vi "guangzi.vi"() -> ()   [LabVIEW 2016]
uses:
  <vilib>/Utility/file.llb/Write To Spreadsheet File (DBL).vi
panel:
  out "切片图":u32[](graph)
  in  "切片值":i32
  in  "选项卡控件":T1(tab)
  in  "对数":bool
  out "MCS8Dat Error":i32
  out "CHN Status":T2 {"Dummy" format="%.2f"; "Starts" format="%.2f"; "Sweeps" format="%.2f"; "Roirate" format="%.2f"; "RoiSum" format="%.2f"; "TotalSum" format="%.2f"; "Fifo full" format="%.2f"; "Runtime" format="%.2f"}
  out "Data":u32[](graph)
  out "Settings":T3 {"dummy3" format="%.2f"; "dummy2" format="%.2f"; "bitshift" format="%.0x"; "Active" format="%.0x"; "Offset" format="%.0x"; "Param" format="%.0x"; "dummy1" format="%.2f"; "Roipreset" format="%.2f"; "cftfak" format="%.0x"}
  out "通道数":i32
  out "Data 9":dbl[](graph)
  out "Data 2":u32[](graph)
  out "MCS8Dat Error 2":i32
  out "Settings 2":T3 {"dummy3" format="%.2f"; "dummy2" format="%.2f"; "bitshift" format="%.0x"; "Active" format="%.0x"; "Offset" format="%.0x"; "Param" format="%.0x"; "dummy1" format="%.2f"; "Roipreset" format="%.2f"; "cftfak" format="%.0x"}
  out "CHN Status 2":T2 {"Dummy" format="%.2f"; "Starts" format="%.2f"; "Sweeps" format="%.2f"; "Roirate" format="%.2f"; "RoiSum" format="%.2f"; "TotalSum" format="%.2f"; "Fifo full" format="%.2f"; "Runtime" format="%.2f"}
  out "通道数 2":i32
  in  "对数 2":bool
  out "Data10":dbl[](graph)
  out "Data 3":u32[](graph)
  out "MCS8Dat Error 3":i32
  out "Settings 3":T3 {"dummy3" format="%.2f"; "dummy2" format="%.2f"; "bitshift" format="%.0x"; "Active" format="%.0x"; "Offset" format="%.0x"; "Param" format="%.0x"; "dummy1" format="%.2f"; "Roipreset" format="%.2f"; "cftfak" format="%.0x"}
  out "CHN Status 3":T2 {"Dummy" format="%.2f"; "Starts" format="%.2f"; "Sweeps" format="%.2f"; "Roirate" format="%.2f"; "RoiSum" format="%.2f"; "TotalSum" format="%.2f"; "Fifo full" format="%.2f"; "Runtime" format="%.2f"}
  out "通道数 3":i32
  in  "对数 3":bool
  out "Data10 2":dbl[](graph)
  out "Data 4":u32[](graph)
  out "MCS8Dat Error 4":i32
  out "Settings 4":T3 {"dummy3" format="%.2f"; "dummy2" format="%.2f"; "bitshift" format="%.0x"; "Active" format="%.0x"; "Offset" format="%.0x"; "Param" format="%.0x"; "dummy1" format="%.2f"; "Roipreset" format="%.2f"; "cftfak" format="%.0x"}
  out "CHN Status 4":T2 {"Dummy" format="%.2f"; "Starts" format="%.2f"; "Sweeps" format="%.2f"; "Roirate" format="%.2f"; "RoiSum" format="%.2f"; "TotalSum" format="%.2f"; "Fifo full" format="%.2f"; "Runtime" format="%.2f"}
  out "通道数 4":i32
  in  "对数 4":bool
  out "Data10 3":dbl[](graph)
  out "Data 5":u32[](graph)
  out "MCS8Dat Error 5":i32
  out "Settings 5":T3 {"dummy3" format="%.2f"; "dummy2" format="%.2f"; "bitshift" format="%.0x"; "Active" format="%.0x"; "Offset" format="%.0x"; "Param" format="%.0x"; "dummy1" format="%.2f"; "Roipreset" format="%.2f"; "cftfak" format="%.0x"}
  out "CHN Status 5":T2 {"Dummy" format="%.2f"; "Starts" format="%.2f"; "Sweeps" format="%.2f"; "Roirate" format="%.2f"; "RoiSum" format="%.2f"; "TotalSum" format="%.2f"; "Fifo full" format="%.2f"; "Runtime" format="%.2f"}
  out "通道数 5":i32
  in  "对数 5":bool
  out "Data10 4":dbl[](graph)
  out "Data 6":u32[](graph)
  out "MCS8Dat Error 6":i32
  out "Settings 6":T3 {"dummy3" format="%.2f"; "dummy2" format="%.2f"; "bitshift" format="%.0x"; "Active" format="%.0x"; "Offset" format="%.0x"; "Param" format="%.0x"; "dummy1" format="%.2f"; "Roipreset" format="%.2f"; "cftfak" format="%.0x"}
  out "CHN Status 6":T2 {"Dummy" format="%.2f"; "Starts" format="%.2f"; "Sweeps" format="%.2f"; "Roirate" format="%.2f"; "RoiSum" format="%.2f"; "TotalSum" format="%.2f"; "Fifo full" format="%.2f"; "Runtime" format="%.2f"}
  out "通道数 6":i32
  in  "对数 6":bool
  out "Data10 5":dbl[](graph)
  out "Data 7":u32[](graph)
  out "MCS8Dat Error 7":i32
  out "Settings 7":T3 {"dummy3" format="%.2f"; "dummy2" format="%.2f"; "bitshift" format="%.0x"; "Active" format="%.0x"; "Offset" format="%.0x"; "Param" format="%.0x"; "dummy1" format="%.2f"; "Roipreset" format="%.2f"; "cftfak" format="%.0x"}
  out "CHN Status 7":T2 {"Dummy" format="%.2f"; "Starts" format="%.2f"; "Sweeps" format="%.2f"; "Roirate" format="%.2f"; "RoiSum" format="%.2f"; "TotalSum" format="%.2f"; "Fifo full" format="%.2f"; "Runtime" format="%.2f"}
  out "通道数 7":i32
  in  "对数 7":bool
  out "Data10 6":dbl[](graph)
  out "Data 8":u32[](graph)
  out "MCS8Dat Error 8":i32
  out "Settings 8":T3 {"dummy3" format="%.2f"; "dummy2" format="%.2f"; "bitshift" format="%.0x"; "Active" format="%.0x"; "Offset" format="%.0x"; "Param" format="%.0x"; "dummy1" format="%.2f"; "Roipreset" format="%.2f"; "cftfak" format="%.0x"}
  out "CHN Status 8":T2 {"Dummy" format="%.2f"; "Starts" format="%.2f"; "Sweeps" format="%.2f"; "Roirate" format="%.2f"; "RoiSum" format="%.2f"; "TotalSum" format="%.2f"; "Fifo full" format="%.2f"; "Runtime" format="%.2f"}
  out "通道数 8":i32
  in  "对数 8":bool
  out "Data10 7":dbl[](graph)
  in  "子开关":bool
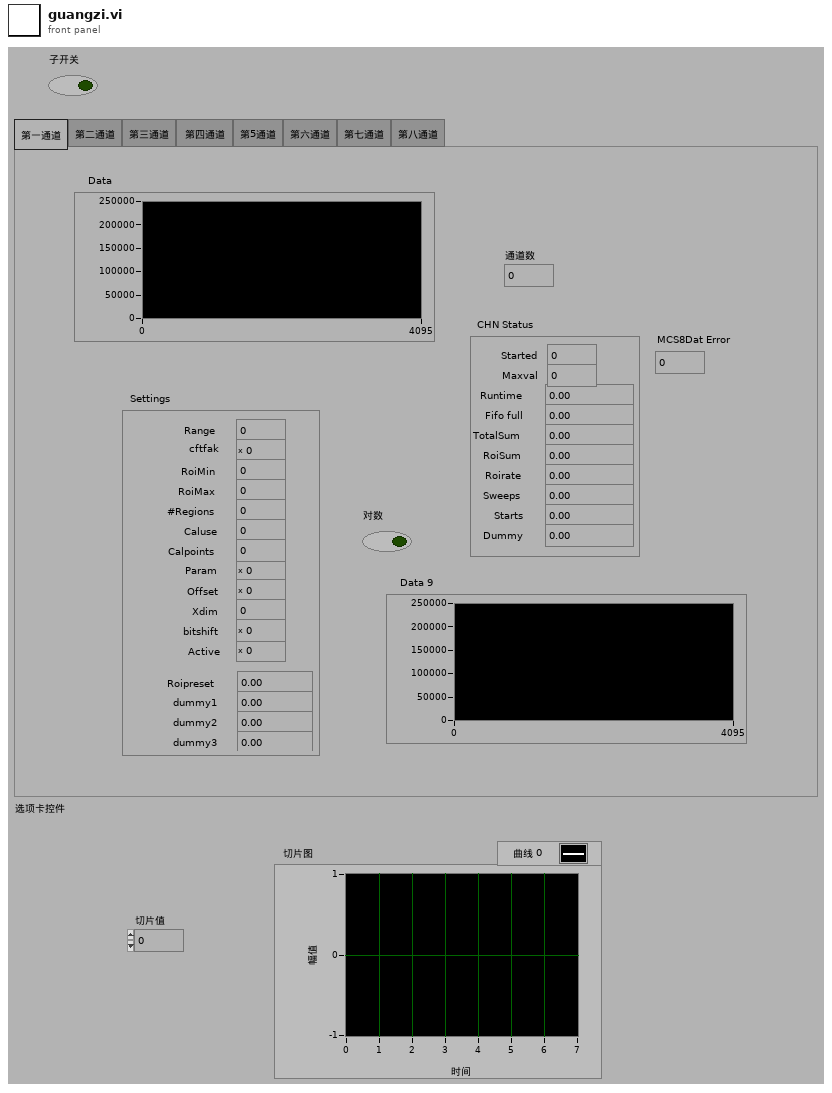
[diagram p1: front panel]
types:
  T1 = enum32{"第一通道", "第二通道", "第三通道", "第四通道 ", "第5通道", "第六通道", "第七通道", "第八通道"}
  T2 = cluster{"Started":i32, "Maxval":u32, "Runtime":dbl, "Fifo full":dbl, "TotalSum":dbl, "RoiSum":dbl, "Roirate":dbl, "Sweeps":dbl, "Starts":dbl, "Dummy":dbl}
  T3 = cluster{"Range":i32, "cftfak":i32, "RoiMin":i32, "RoiMax":i32, "#Regions":i32, "Caluse":i32, "Calpoints":i32, "Param":i32, "Offset":i32, "Xdim":i32, "bitshift":i32, "Active":i32, "Roipreset":dbl, "dummy1":dbl, "dummy2":dbl, "dummy3":dbl}
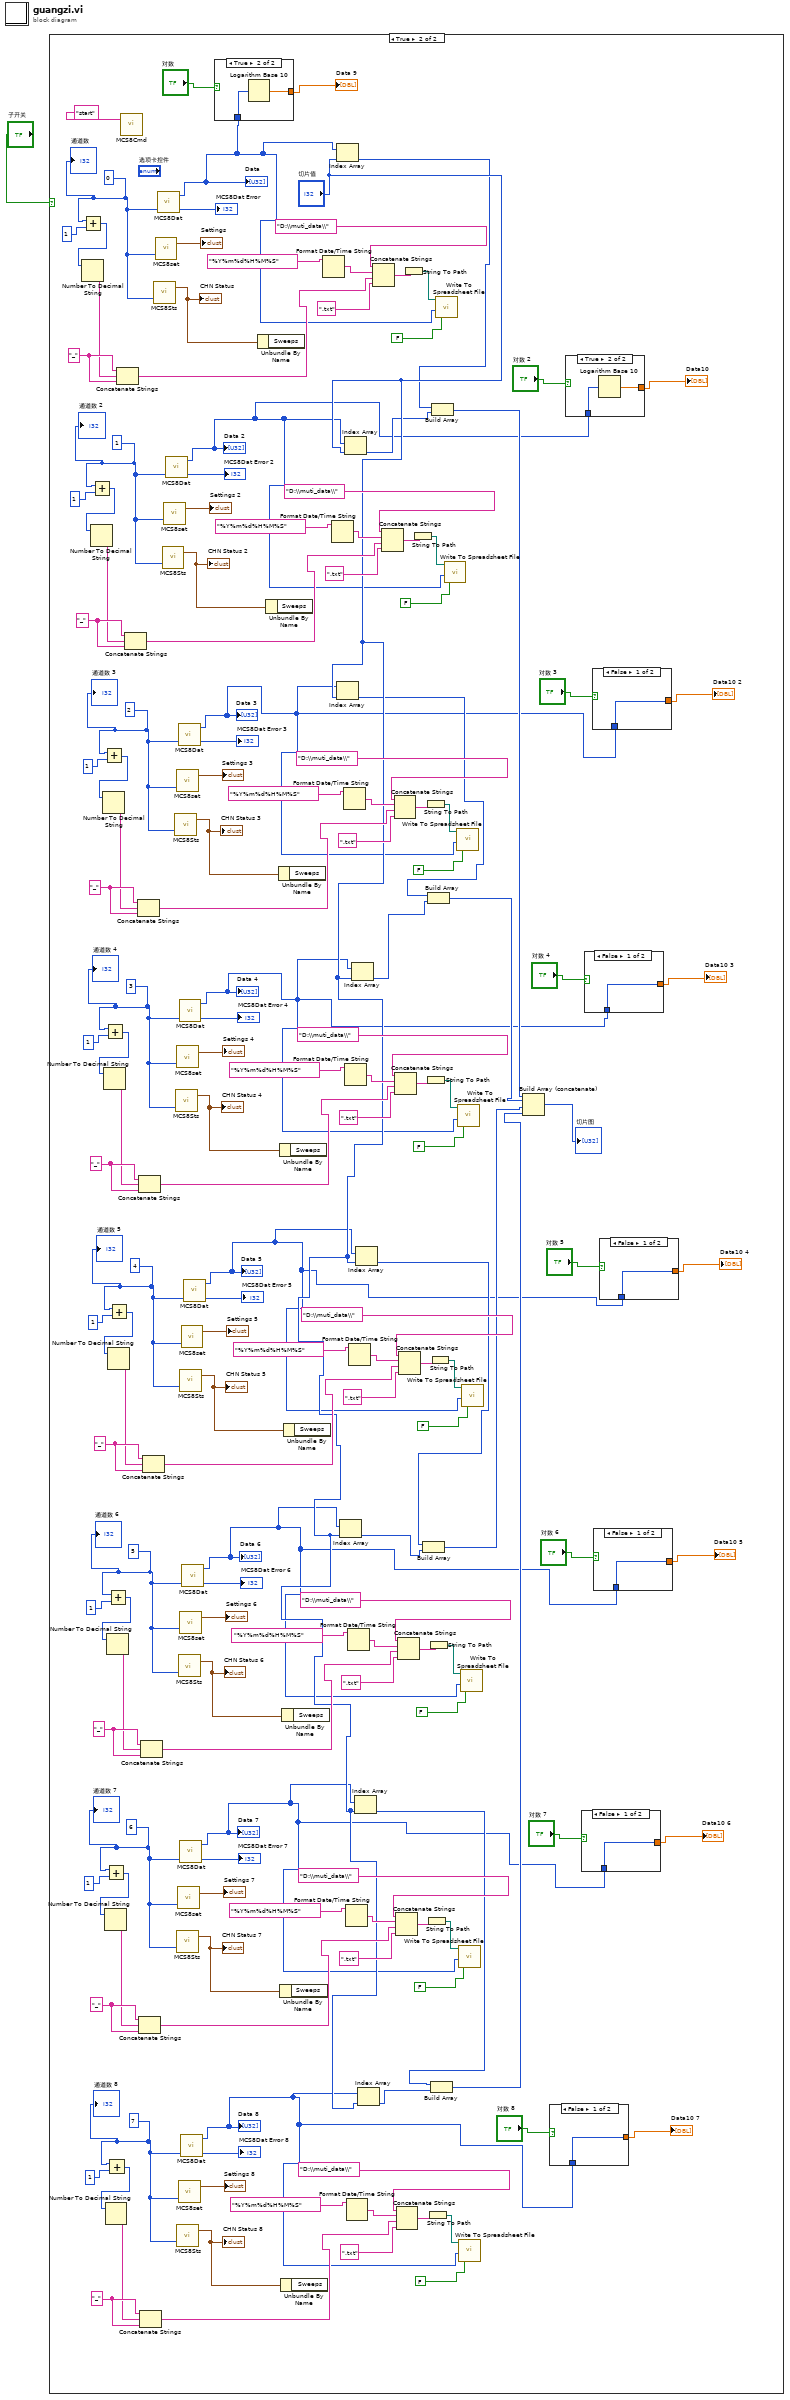
[diagram p0: block diagram]
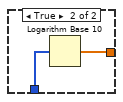
[diagram p3: hidden frame]
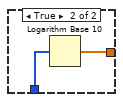
[diagram p4: hidden frame]
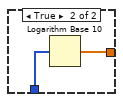
[diagram p5: hidden frame]
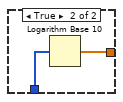
[diagram p6: hidden frame]
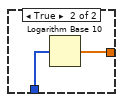
[diagram p7: hidden frame]
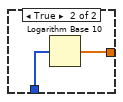
[diagram p8: hidden frame]
diagram:
  n1 = case shown="True" "子开关" {
    frame False {
    }
    frame True {
      w40 = 7
      w49 = "_"
      w56 = 6
      w65 = "_"
      w72 = 5
      w81 = "_"
      w88 = 4
      w97 = "_"
      w104 = 3
      w113 = "_"
      w120 = 2
      w129 = "_"
      w136 = 1
      w145 = "_"
      w152 = 0
      w161 = "_"
      n2 = Add(x=w152, y=1) -> (x+y=w155:i32)
      n3 = Number To Decimal String(number=w155) -> (decimal integer string=w160:string)  [unwired: 1 in]
      n4 = Add(x=w136, y=1) -> (x+y=w139:i32)
      n5 = Number To Decimal String(number=w139) -> (decimal integer string=w144:string)  [unwired: 1 in]
      n6 = Add(x=w120, y=1) -> (x+y=w123:i32)
      n7 = Number To Decimal String(number=w123) -> (decimal integer string=w128:string)  [unwired: 1 in]
      n8 = Add(x=w104, y=1) -> (x+y=w107:i32)
      n9 = Number To Decimal String(number=w107) -> (decimal integer string=w112:string)  [unwired: 1 in]
      n10 = Add(x=w56, y=1) -> (x+y=w59:i32)
      n11 = Number To Decimal String(number=w59) -> (decimal integer string=w64:string)  [unwired: 1 in]
      n12 = Add(x=w40, y=1) -> (x+y=w43:i32)
      n13 = Number To Decimal String(number=w43) -> (decimal integer string=w48:string)  [unwired: 1 in]
      n14 = Add(x=w72, y=1) -> (x+y=w75:i32)
      n15 = Number To Decimal String(number=w75) -> (decimal integer string=w80:string)  [unwired: 1 in]
      n16 = Add(x=w88, y=1) -> (x+y=w91:i32)
      n17 = Number To Decimal String(number=w91) -> (decimal integer string=w96:string)  [unwired: 1 in]
      n18 = Concatenate Strings(w161, w160, w161) -> (w159:string)
      n19 = call "MCS8Cmd.vi"("Command"="start") -> ()  [unwired: 2 in, 1 out]
      n20 = Concatenate Strings(w145, w144, w145) -> (w143:string)
      n21 = Concatenate Strings(w129, w128, w129) -> (w127:string)
      n22 = Concatenate Strings(w113, w112, w113) -> (w111:string)
      n23 = Concatenate Strings(w65, w64, w65) -> (w63:string)
      n24 = Concatenate Strings(w49, w48, w49) -> (w47:string)
      n25 = Concatenate Strings(w81, w80, w81) -> (w79:string)
      n26 = Concatenate Strings(w97, w96, w97) -> (w95:string)
      n27 = call "MCS8Sts.vi"("CHN #"=w152) -> ("CHN Status"=w167:T2)  [unwired: 1 in, 1 out]
      "CHN Status" <- w167
      n28 = call "MCS8set.vi"("Spect #"=w152) -> ("Settings"=→"Settings":T3)  [unwired: 1 in, 1 out]
      n29 = call "MCS8Dat.vi"("Spectrum #"=w152) -> ("MCS8Dat Error"=→"MCS8Dat Error":i32, "Data"=w24:u32[])  [unwired: 2 in, 1 out]
      "Data" <- w24
      n30 = call "MCS8Sts.vi"("CHN #"=w136) -> ("CHN Status"=w151:T2)  [unwired: 1 in, 1 out]
      "CHN Status 2" <- w151
      n31 = call "MCS8set.vi"("Spect #"=w136) -> ("Settings"=→"Settings 2":T3)  [unwired: 1 in, 1 out]
      n32 = call "MCS8Dat.vi"("Spectrum #"=w136) -> ("MCS8Dat Error"=→"MCS8Dat Error 2":i32, "Data"=w20:u32[])  [unwired: 2 in, 1 out]
      "Data 2" <- w20
      n33 = call "MCS8Sts.vi"("CHN #"=w120) -> ("CHN Status"=w135:T2)  [unwired: 1 in, 1 out]
      "CHN Status 3" <- w135
      n34 = call "MCS8Sts.vi"("CHN #"=w104) -> ("CHN Status"=w119:T2)  [unwired: 1 in, 1 out]
      "CHN Status 4" <- w119
      n35 = call "MCS8set.vi"("Spect #"=w120) -> ("Settings"=→"Settings 3":T3)  [unwired: 1 in, 1 out]
      n36 = call "MCS8Sts.vi"("CHN #"=w56) -> ("CHN Status"=w71:T2)  [unwired: 1 in, 1 out]
      "CHN Status 7" <- w71
      n37 = call "MCS8set.vi"("Spect #"=w104) -> ("Settings"=→"Settings 4":T3)  [unwired: 1 in, 1 out]
      n38 = call "MCS8Sts.vi"("CHN #"=w40) -> ("CHN Status"=w55:T2)  [unwired: 1 in, 1 out]
      "CHN Status 8" <- w55
      n39 = call "MCS8set.vi"("Spect #"=w56) -> ("Settings"=→"Settings 7":T3)  [unwired: 1 in, 1 out]
      n40 = call "MCS8Dat.vi"("Spectrum #"=w120) -> ("MCS8Dat Error"=→"MCS8Dat Error 3":i32, "Data"=w17:u32[])  [unwired: 2 in, 1 out]
      "Data 3" <- w17
      n41 = call "MCS8Sts.vi"("CHN #"=w72) -> ("CHN Status"=w87:T2)  [unwired: 1 in, 1 out]
      "CHN Status 6" <- w87
      n42 = call "MCS8set.vi"("Spect #"=w40) -> ("Settings"=→"Settings 8":T3)  [unwired: 1 in, 1 out]
      n43 = call "MCS8Dat.vi"("Spectrum #"=w104) -> ("MCS8Dat Error"=→"MCS8Dat Error 4":i32, "Data"=w14:u32[])  [unwired: 2 in, 1 out]
      "Data 4" <- w14
      n44 = call "MCS8Sts.vi"("CHN #"=w88) -> ("CHN Status"=w103:T2)  [unwired: 1 in, 1 out]
      "CHN Status 5" <- w103
      n45 = call "MCS8set.vi"("Spect #"=w72) -> ("Settings"=→"Settings 6":T3)  [unwired: 1 in, 1 out]
      n46 = call "MCS8Dat.vi"("Spectrum #"=w56) -> ("MCS8Dat Error"=→"MCS8Dat Error 7":i32, "Data"=w5:u32[])  [unwired: 2 in, 1 out]
      "Data 7" <- w5
      n47 = call "MCS8Dat.vi"("Spectrum #"=w40) -> ("MCS8Dat Error"=→"MCS8Dat Error 8":i32, "Data"=w2:u32[])  [unwired: 2 in, 1 out]
      "Data 8" <- w2
      n48 = call "MCS8set.vi"("Spect #"=w88) -> ("Settings"=→"Settings 5":T3)  [unwired: 1 in, 1 out]
      n49 = call "MCS8Dat.vi"("Spectrum #"=w72) -> ("MCS8Dat Error"=→"MCS8Dat Error 6":i32, "Data"=w8:u32[])  [unwired: 2 in, 1 out]
      "Data 6" <- w8
      n50 = call "MCS8Dat.vi"("Spectrum #"=w88) -> ("MCS8Dat Error"=→"MCS8Dat Error 5":i32, "Data"=w11:u32[])  [unwired: 2 in, 1 out]
      "Data 5" <- w11
      n51 = case shown="True" "对数" {
        tunnel: w24 -> [w190 w192]
        tunnel: [w190 w191] -> w23
        frame False {
        }
        frame True {
          n52 = Logarithm Base 10(1:w192) -> (0:w191:dbl[])
        }
      }
      "Data 9" <- w23
      n53 = Unbundle By Name(w167) -> ()  [unwired: 1 out]
      n54 = Unbundle By Name(w151) -> ()  [unwired: 1 out]
      n55 = Unbundle By Name(w135) -> ()  [unwired: 1 out]
      n56 = Unbundle By Name(w119) -> ()  [unwired: 1 out]
      n57 = Unbundle By Name(w71) -> ()  [unwired: 1 out]
      n58 = Unbundle By Name(w55) -> ()  [unwired: 1 out]
      n59 = Unbundle By Name(w87) -> ()  [unwired: 1 out]
      n60 = Unbundle By Name(w103) -> ()  [unwired: 1 out]
      n61 = Format Date/Time String(time format string (%c)="%Y%m%d%H%M%S") -> (date/time string=w156:string)  [unwired: 2 in]
      n62 = Format Date/Time String(time format string (%c)="%Y%m%d%H%M%S") -> (date/time string=w140:string)  [unwired: 2 in]
      n63 = Index Array(array=w24, index="切片值") -> (element=w32:u32)
      n64 = Index Array(array=w17, index="切片值") -> (element=w34:u32)
      n65 = Index Array(array=w8, index="切片值") -> (element=w36:u32)
      n66 = Format Date/Time String(time format string (%c)="%Y%m%d%H%M%S") -> (date/time string=w124:string)  [unwired: 2 in]
      n67 = Index Array(array=w20, index="切片值") -> (element=w31:u32)
      n68 = Format Date/Time String(time format string (%c)="%Y%m%d%H%M%S") -> (date/time string=w108:string)  [unwired: 2 in]
      n69 = Format Date/Time String(time format string (%c)="%Y%m%d%H%M%S") -> (date/time string=w60:string)  [unwired: 2 in]
      n70 = Format Date/Time String(time format string (%c)="%Y%m%d%H%M%S") -> (date/time string=w44:string)  [unwired: 2 in]
      n71 = Format Date/Time String(time format string (%c)="%Y%m%d%H%M%S") -> (date/time string=w76:string)  [unwired: 2 in]
      n72 = Format Date/Time String(time format string (%c)="%Y%m%d%H%M%S") -> (date/time string=w92:string)  [unwired: 2 in]
      n73 = Index Array(array=w14, index="切片值") -> (element=w33:u32)
      n74 = Index Array(array=w5, index="切片值") -> (element=w37:u32)
      n75 = Index Array(array=w11, index="切片值") -> (element=w35:u32)
      n76 = Index Array(array=w2, index="切片值") -> (element=w38:u32)
      n77 = Concatenate Strings("D:\\muti_data\\", w156, w159, ".txt") -> (w164:string)
      n78 = Concatenate Strings("D:\\muti_data\\", w140, w143, ".txt") -> (w148:string)
      n79 = Concatenate Strings("D:\\muti_data\\", w124, w127, ".txt") -> (w132:string)
      n80 = Concatenate Strings("D:\\muti_data\\", w108, w111, ".txt") -> (w116:string)
      n81 = Concatenate Strings("D:\\muti_data\\", w60, w63, ".txt") -> (w68:string)
      n82 = Concatenate Strings("D:\\muti_data\\", w44, w47, ".txt") -> (w52:string)
      n83 = Concatenate Strings("D:\\muti_data\\", w76, w79, ".txt") -> (w84:string)
      n84 = Concatenate Strings("D:\\muti_data\\", w92, w95, ".txt") -> (w100:string)
      n85 = String To Path(string=w164) -> (path=w163:path)
      n86 = String To Path(string=w148) -> (path=w147:path)
      n87 = Build Array(w35, w36) -> (w28:u32[])
      n88 = String To Path(string=w132) -> (path=w131:path)
      n89 = String To Path(string=w116) -> (path=w115:path)
      n90 = String To Path(string=w68) -> (path=w67:path)
      n91 = String To Path(string=w52) -> (path=w51:path)
      n92 = Build Array(w34, w33) -> (w29:u32[])
      n93 = String To Path(string=w84) -> (path=w83:path)
      n94 = String To Path(string=w100) -> (path=w99:path)
      n95 = Build Array(w37, w38) -> (w27:u32[])
      n96 = Build Array(w32, w31) -> (w30:u32[])
      n97 = call-poly <vilib>:"Write To Spreadsheet File.vi"("append to file? (new file:F)"=FALSE, "1D data"=w24, "file path (dialog if empty)"=w163) -> ()  [unwired: 5 in, 1 out]
      n98 = call-poly <vilib>:"Write To Spreadsheet File.vi"("append to file? (new file:F)"=FALSE, "1D data"=w20, "file path (dialog if empty)"=w147) -> ()  [unwired: 5 in, 1 out]
      n99 = call-poly <vilib>:"Write To Spreadsheet File.vi"("append to file? (new file:F)"=FALSE, "1D data"=w17, "file path (dialog if empty)"=w131) -> ()  [unwired: 5 in, 1 out]
      n100 = call-poly <vilib>:"Write To Spreadsheet File.vi"("append to file? (new file:F)"=FALSE, "1D data"=w14, "file path (dialog if empty)"=w115) -> ()  [unwired: 5 in, 1 out]
      n101 = call-poly <vilib>:"Write To Spreadsheet File.vi"("append to file? (new file:F)"=FALSE, "1D data"=w5, "file path (dialog if empty)"=w67) -> ()  [unwired: 5 in, 1 out]
      n102 = call-poly <vilib>:"Write To Spreadsheet File.vi"("append to file? (new file:F)"=FALSE, "1D data"=w2, "file path (dialog if empty)"=w51) -> ()  [unwired: 5 in, 1 out]
      n103 = call-poly <vilib>:"Write To Spreadsheet File.vi"("append to file? (new file:F)"=FALSE, "1D data"=w8, "file path (dialog if empty)"=w83) -> ()  [unwired: 5 in, 1 out]
      n104 = call-poly <vilib>:"Write To Spreadsheet File.vi"("append to file? (new file:F)"=FALSE, "1D data"=w11, "file path (dialog if empty)"=w99) -> ()  [unwired: 5 in, 1 out]
      n105 = Build Array (concatenate)(w30, w29, w28, w27) -> (→"切片图":u32[])
      n106 = case shown="False" "对数 8" {
        tunnel: w2 -> [w169 w171]
        tunnel: [w169 w170] -> w3
        frame False {
        }
        frame True {
          n107 = Logarithm Base 10(1:w171) -> (0:w170:dbl[])
        }
      }
      "Data10 7" <- w3
      n108 = case shown="True" "对数 2" {
        tunnel: w20 -> [w187 w189]
        tunnel: [w187 w188] -> w21
        frame False {
        }
        frame True {
          n109 = Logarithm Base 10(1:w189) -> (0:w188:dbl[])
        }
      }
      "Data10" <- w21
      n110 = case shown="False" "对数 7" {
        tunnel: w5 -> [w172 w174]
        tunnel: [w172 w173] -> w6
        frame False {
        }
        frame True {
          n111 = Logarithm Base 10(1:w174) -> (0:w173:dbl[])
        }
      }
      "Data10 6" <- w6
      n112 = case shown="False" "对数 4" {
        tunnel: w14 -> [w181 w183]
        tunnel: [w181 w182] -> w15
        frame False {
        }
        frame True {
          n113 = Logarithm Base 10(1:w183) -> (0:w182:dbl[])
        }
      }
      "Data10 3" <- w15
      n114 = case shown="False" "对数 3" {
        tunnel: w17 -> [w184 w186]
        tunnel: [w184 w185] -> w18
        frame False {
        }
        frame True {
          n115 = Logarithm Base 10(1:w186) -> (0:w185:dbl[])
        }
      }
      "Data10 2" <- w18
      n116 = case shown="False" "对数 6" {
        tunnel: w8 -> [w175 w177]
        tunnel: [w175 w176] -> w9
        frame False {
        }
        frame True {
          n117 = Logarithm Base 10(1:w177) -> (0:w176:dbl[])
        }
      }
      "Data10 5" <- w9
      n118 = case shown="False" "对数 5" {
        tunnel: w11 -> [w178 w180]
        tunnel: [w178 w179] -> w12
        frame False {
        }
        frame True {
          n119 = Logarithm Base 10(1:w180) -> (0:w179:dbl[])
        }
      }
      "Data10 4" <- w12
      "通道数" <- w152
      "通道数 2" <- w136
      "通道数 3" <- w120
      "通道数 4" <- w104
      "通道数 5" <- w88
      "通道数 6" <- w72
      "通道数 7" <- w56
      "通道数 8" <- w40
    }
  }
